vi "SCADA Plataforma_v3.vi"() -> ()   [LabVIEW 2020]
uses:
  <vilib>/Instr/_visa.llb/VISA Configure Serial Port (Instr).vi
panel:
  out "REACTION WHEEL Y":bool
  in  "Tab Control 5":enum32{"YAW", "GYRO Z", "ACC Z"}(tab)
  out "CUBESAT'S YAW ANGLE":sgl[](graph)
  out "CUBESAT'S Z ANGULAR RATE":sgl[](graph)
  out "CUBESAT'S ACCELERATION IN Z":sgl[](graph)
  in  "Tab Control 4":enum32{"PITCH", "GIRO Y", "ACC Y"}(tab)
  out "CUBESAT'S PITCH ANGLE":sgl[](graph)
  out "CUBESAT'S Y ANGULAR RATE":sgl[](graph)
  out "CUBESAT'S ACCELERATION IN Y":sgl[](graph)
  in  "Tab Control 3":enum32{"ROLL", "GYRO X", "ACC X"}(tab)
  out "CUBESAT'S ROLL ANGLE":sgl[](graph)
  out "CUBESAT'S X ANGULAR RATE":sgl[](graph)
  out "CUBESAT'S ACCELERATION IN X":sgl[](graph)
  in  "Tab Control 2":enum32{"RW X", "RW Y", "RW Z"}(tab)
  out "REACTION WHEEL X CURRENT":dbl[](graph)
  out "REACTION WHEEL Y CURRENT":dbl[](graph)
  out "REACTION WHEEL Z CURRENT":dbl[](graph)
  in  "Tab Control":enum32{"RW X", "RW Y", "RW Z"}(tab)
  out "REACTION WHEEL X RATE":sgl[](graph)
  out "REACTION WHEEL Y RATE":sgl[](graph)
  out "REACTION WHEEL Z RATE":sgl[](graph)
  out "Rate 3":dbl
  in  "RWZ - Duty Cicle (PWM)":u16(knob) max=4999 step=1 scale=0.0..4999.0
  in  "RW3 Direction":bool
  out "REACTION WHEEL Z":bool
  out "Rate 2":dbl
  in  "RWY - Duty Cicle (PWM)":u16(knob) max=4999 step=1 scale=0.0..4999.0
  in  "RW2 Direction":bool
  out "Rate 1":dbl
  in  "RW X - Duty Cicle (PWM)":u16(knob) max=4999 step=1 scale=0.0..4999.0
  in  "RW1 Direction":bool
  out "REACTION WHEEL X":bool
  in  "ActiveX Container 7":refnum<k7>(container)
  in  "SET:":bool
  in  "ON  /  OFF":bool
  in  "ActiveX Container 5":refnum<k7>(container)
  in  "ActiveX Container 4":refnum<k7>(container)
  out "Recepción":bool
  out "Transmisión":bool
  in  "Incomming Bytes:":u32
  in  "PORT:":refnum<visa-resource-name>
  in  "Baud Rate:":u32=9600
  in  "ActiveX Container 2":refnum<k7>(container)
  in  "PARADA DE EMERGENCIA":bool
  in  "ActiveX Container":refnum<k7>(container)
  # "Test platform for attitude determination and control of \nUNSat I"
  # "SETTINGS"
  # "MANUAL CONTROL"
  # "REACTION WHEELS SETTINGS"
  # "Encoder Resolution:"
  # "CCW"
  # "CW"
  # "CCW"
  # "CW"
  # "CCW"
  # "CW"
  # "DEVELOPED BY:"
  # "Hammerly Mamani Valencia"
  # "Modified by:"
  # "Brayan Espinoza"
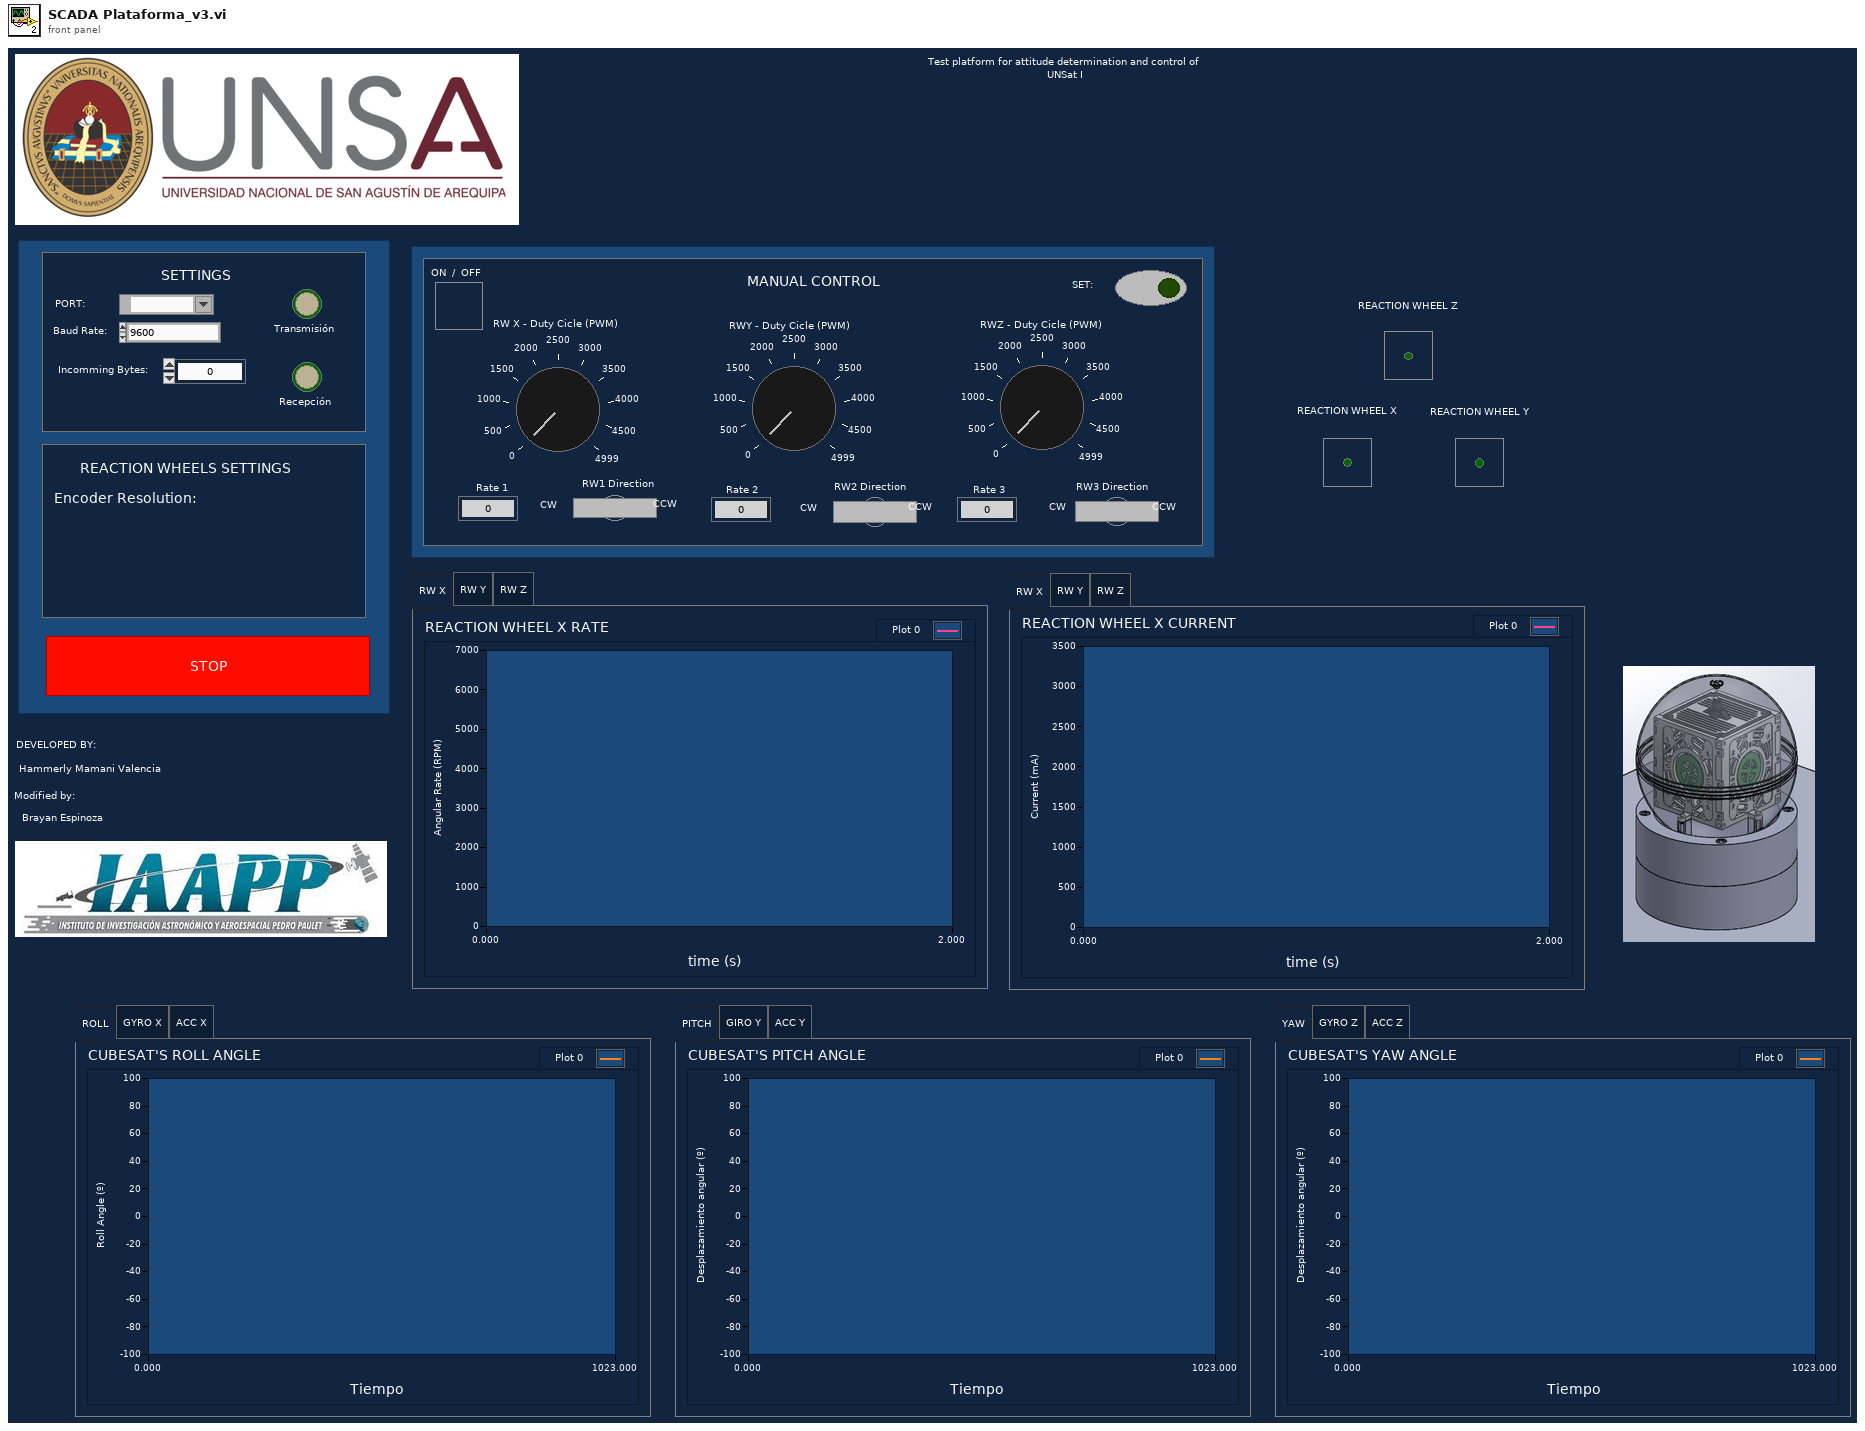
[diagram p1: front panel]
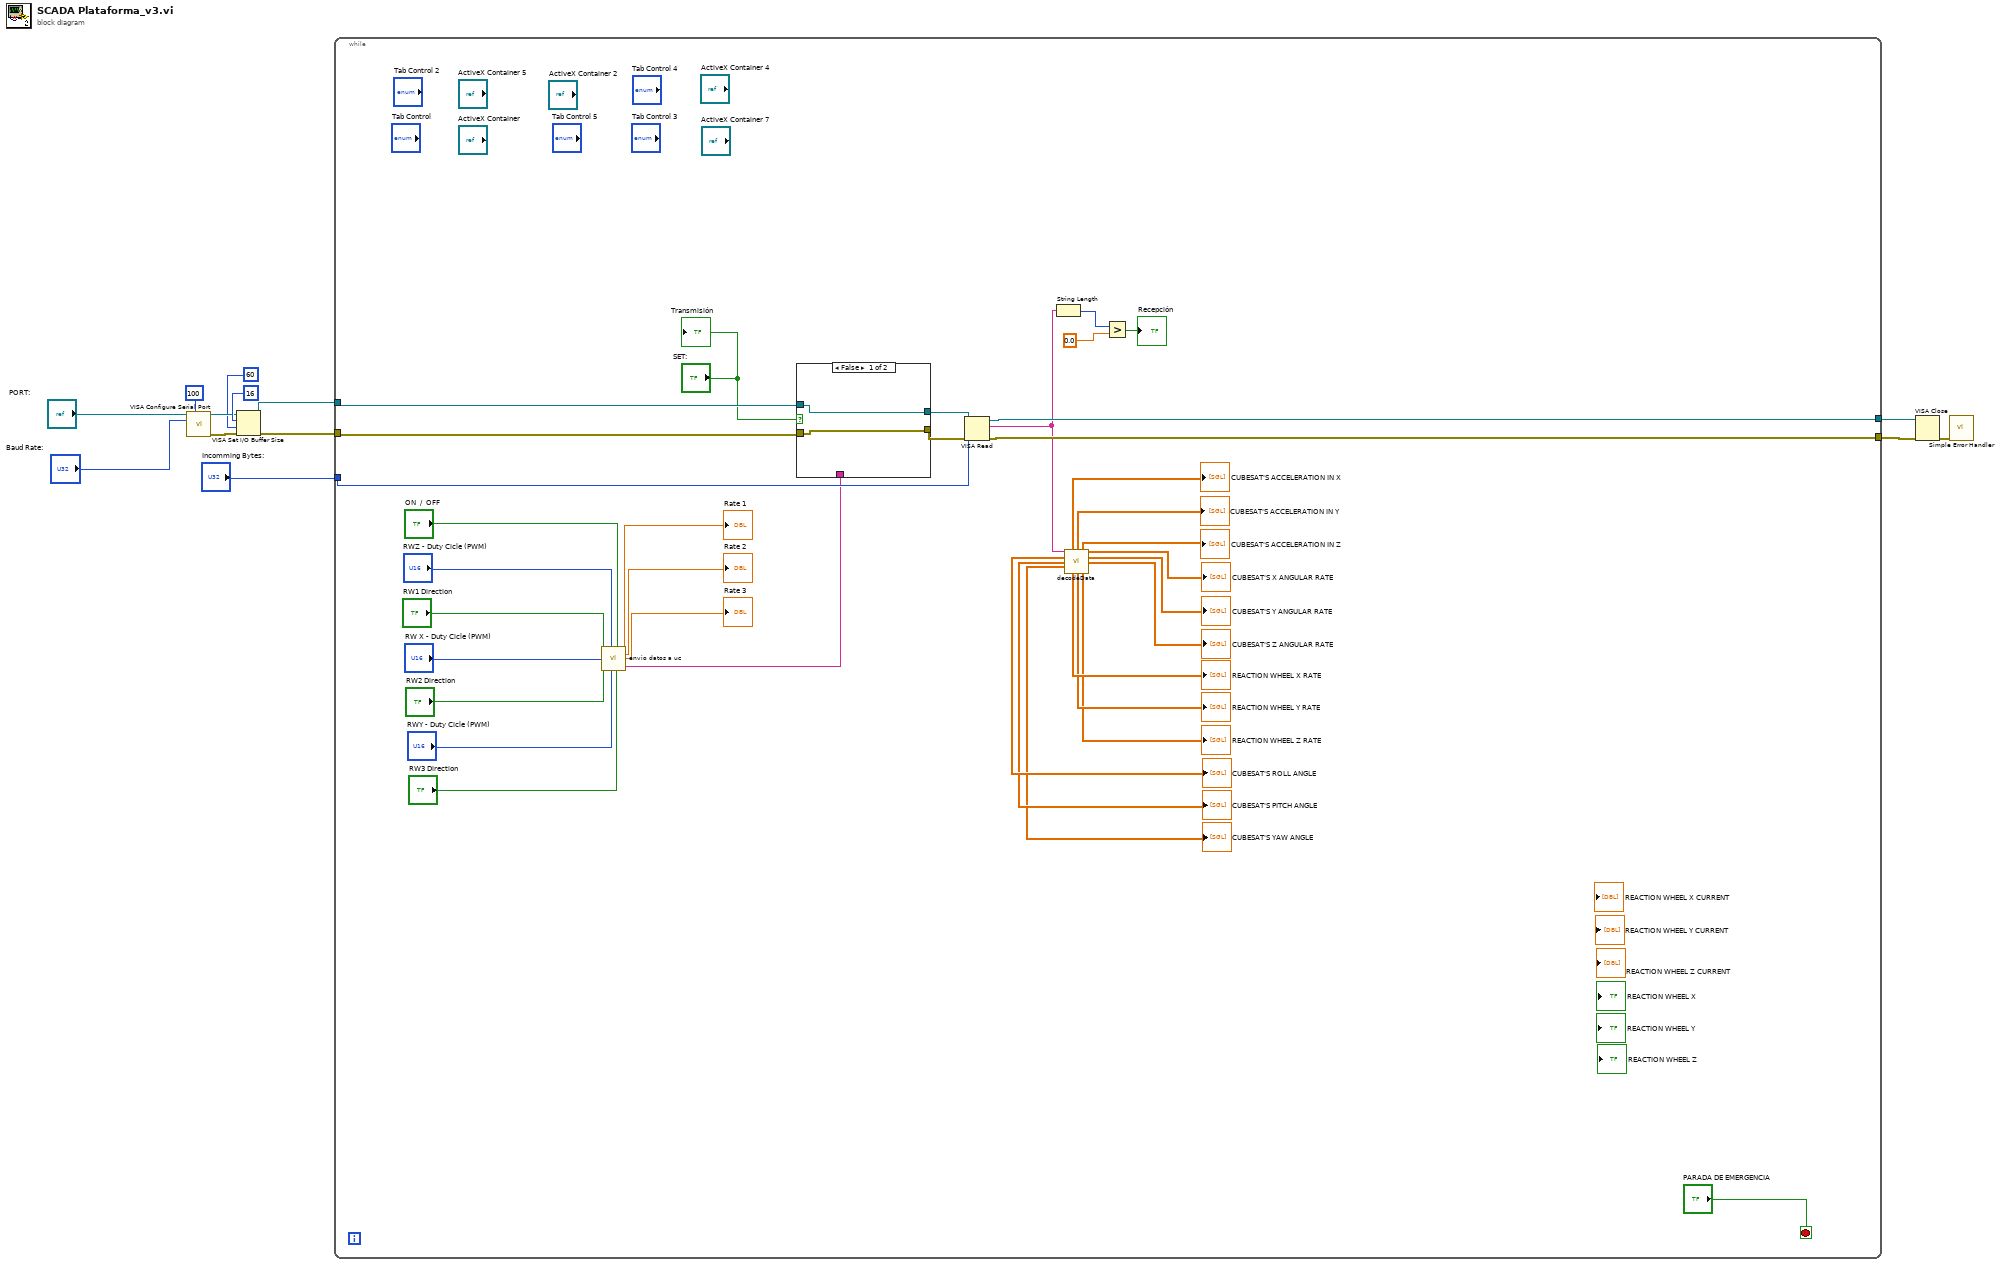
[diagram p0: block diagram]
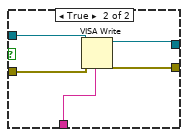
[diagram p2: hidden frame]
diagram:
  n1 = call-poly "VISA Configure Serial Port"("VISA resource name"="PORT:", "timeout (10sec)"=u32 100, "baud rate (9600)"="Baud Rate:") -> ("VISA resource name out"=w8:refnum<visa-resource-name>, "error out"=w7:errorcluster)  [unwired: 11 in]
  n2 = VISA Set I/O Buffer Size(VISA resource name=w8, mask (16)=u16 16 ("I/O Receive\nBuffer mask"), size (4096)=u32 60, error in (no error)=w7) -> (VISA resource name out=w1:refnum<visa-resource-name>, error out=w6:errorcluster)
  n3 = while {
    tunnel: w1 -> [w47]
    tunnel: w6 -> [w32]
    tunnel: [w49] -> w12
    tunnel: [w48] -> w11
    tunnel: "Incomming Bytes:" -> [w39]
    stop <- "PARADA DE EMERGENCIA" stop-if-true
    n4 = call "envio datos a uc.vi"("ON  /  OFF"="ON  /  OFF", "Sentido de Giro 3"="RW3 Direction", "VELOCIDAD (PWM 3- Duty Cicle)"="RWZ - Duty Cicle (PWM)", "Sentido de Giro 2"="RW2 Direction", "VELOCIDAD (PWM 2 - Duty Cicle)"="RWY - Duty Cicle (PWM)", "Sentido de Giro 1"="RW1 Direction", "VELOCIDAD (PWM 1 - Duty Cicle)"="RW X - Duty Cicle (PWM)") -> ("Velocidad 3"=→"Rate 3":dbl, "Velocidad 2"=→"Rate 2":dbl, "Velocidad 1"=→"Rate 1":dbl, "String"=w27:string)
    n5 = case shown="False" "SET:" {
      tunnel: w47 -> [w51 w56]
      tunnel: [w51 w55] -> w46
      tunnel: [w50 w54] -> w45
      tunnel: w32 -> [w50 w53]
      tunnel: w27 -> [_ w52]
      frame False {
      }
      frame True {
        n6 = VISA Write(VISA resource name=w56, write buffer=w52, error in (no error)=w53) -> (VISA resource name out=w55:refnum<visa-resource-name>, error out=w54:errorcluster)  [unwired: 1 out]
      }
    }
    n7 = VISA Read(VISA resource name=w46, byte count=w39, error in (no error)=w45) -> (VISA resource name out=w49:refnum<visa-resource-name>, read buffer=w26:string, error out=w48:errorcluster)  [unwired: 1 out]
    n8 = String Length(string=w26) -> (length=w41:i32)
    n9 = call "decodeData.vi"("Read Buffer"=w26) -> ("Acc X"=→"CUBESAT'S ACCELERATION IN X":sgl[], "AccY"=→"CUBESAT'S ACCELERATION IN Y":sgl[], "AccZ"=→"CUBESAT'S ACCELERATION IN Z":sgl[], "GyroX"=→"CUBESAT'S X ANGULAR RATE":sgl[], "Roll"=→"CUBESAT'S ROLL ANGLE":sgl[], "GyroY"=→"CUBESAT'S Y ANGULAR RATE":sgl[], "Pitch"=→"CUBESAT'S PITCH ANGLE":sgl[], "GyroZ"=→"CUBESAT'S Z ANGULAR RATE":sgl[], "Yaw"=→"CUBESAT'S YAW ANGLE":sgl[], "RwX"=→"REACTION WHEEL X RATE":sgl[], "RwY"=→"REACTION WHEEL Y RATE":sgl[], "RwZ"=→"REACTION WHEEL Z RATE":sgl[])  [unwired: 3 in]
    n10 = Greater?(x=w41, y=0.0) -> (0:→"Recepción":bool)
    "Transmisión" <- "SET:"
  }
  n11 = VISA Close(VISA resource name=w12, error in (no error)=w11) -> (error out=w13:errorcluster)
  n12 = call <vilib>:"Simple Error Handler.vi"("error in (no error)"=w13) -> ()  [unwired: 4 in, 5 out]
